vi "PID Custom.vi"(8 "error in (no error)":errorcluster, 9 "Error Motor B":dbl, 10 "Error Motor A":dbl, 11 "Initialise":bool) -> (0 "error out":errorcluster, 1 "Output 2":dbl, 2 "Output":dbl)   [LabVIEW 2016]
uses:
  <vilib>/Simulation/Scripting/Companion Diagram/SimConfigNode/SimParams.ctl
  <vilib>/Simulation/Scripting/Companion Diagram/SimConfigNode/_simSolvers.ctl
  <vilib>/Simulation/Implementation/Shared/SIMSCR Execution Mode.ctl
  <vilib>/Simulation/Param Hierarchy/Typedefs/SIMPH Param Control Actions.ctl
  <vilib>/Simulation/Implementation/Shared/NILVSim_ParamChanged.vi
  <vilib>/Simulation/Implementation/Shared/NILVSIM_BeginStep.vi
  <vilib>/Simulation/Implementation/Shared/NILVSim_Manager.vi
  <vilib>/Utility/error.llb/Clear Errors.vi
  <vilib>/Simulation/Implementation/Shared/NILVSim_FinalizeModel.vi
  <vilib>/Simulation/Implementation/Shared/SIM Unbundle Sim Info.vi
  <vilib>/Simulation/Implementation/Shared/NILVSim_Initialize.vi
  <vilib>/Simulation/Utility/Implementation/NILVSim Get Time and IsAcceptedStep.vi
  <vilib>/Simulation/Implementation/Shared/SIMSH Read Queue.vi
  <vilib>/Simulation/Implementation/Shared/NILVSim_GetModelError.vi
  <vilib>/Simulation/Implementation/Shared/SIM Bundle Sim Info.vi
  <vilib>/Simulation/Implementation/XNodeFramework/SimXNode/SimX.xnode
  <vilib>/Simulation/Model Libraries/PID/SIM PID (Parallel).vi
  <vilib>/Simulation/Model Libraries/PID/SIM PID.vi
  <vilib>/Simulation/Scripting/Companion Diagram/SimConfigNode/SimDog.xnode
  <vilib>/Simulation/Model Libraries/PID/SIM PID (Academic).vi
  <vilib>/Simulation/Implementation/Shared/NI_SIM_Implementation.lvlib
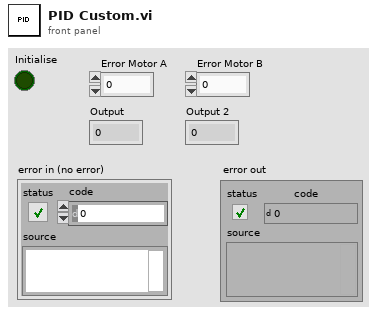
[diagram p1: front panel]
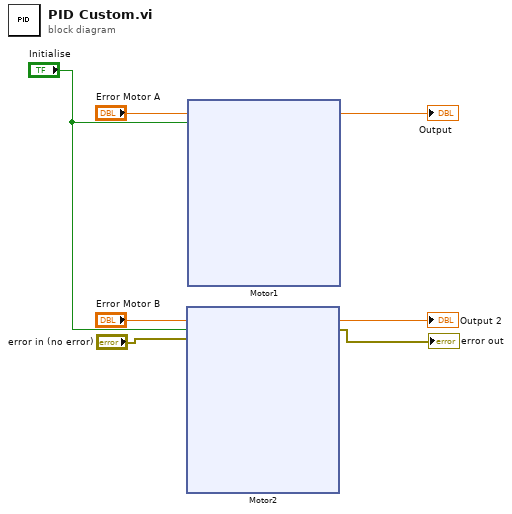
[diagram p0: block diagram]
diagram:
  n1 = xnode "Motor2"("Error"="Error Motor B", "Initialize"="Initialise", "error in"="error in (no error)") -> ("Output"=→"Output 2":dbl, "error out"=→"error out":errorcluster)  [unwired: 10 out]
  n2 = xnode "Motor1"("Error"="Error Motor A", "Initialize"="Initialise") -> ("Output"=→"Output":dbl)  [unwired: 1 in, 11 out]
